vi "Launch Main.vi"(8 "error in":errorcluster, 9 "Name":string, 10 "Path":path=path "C:/Users/Public/Documents/Development/AppDemo", 11 "notifier in":refnum<notifier>) -> (0 "error out":errorcluster, 2 "Main Enqueuer":refnum<class "Message Enqueuer.lvclass">, 3 "notifier out":refnum<notifier>)   [LabVIEW 2023, in "Main.lvlib"]
uses:
  Library/Main.lvlib
  Library/Main.lvclass
  builds/Framework/Panel Manager.lvlibp/Panel/Window Position/Reference Position/Alignment.ctl
  builds/Framework/Panel Manager.lvlibp/Panel/Window Position/Reference Position/Horizontal Alignment.ctl
  builds/Framework/Panel Manager.lvlibp/Panel/Window Position/Reference Position/Vertical Alignment.ctl
  builds/Framework/Panel Manager.lvlibp/Panel/Window Position/Reference Position/Ref Display/Ref Display.lvclass
  builds/Framework/Engine.lvlibp/Engine/Accessors/Write IsRoot.vi
  builds/Framework/Engine.lvlibp/Engine/Accessors/Write Application Path.vi
  builds/Framework/Panel Manager.lvlibp/Panel Actor/Panel Actor/Launch Root Panel Window.vi
  builds/Framework/Panel Manager.lvlibp/Panel/Window Position/Reference Position/Ref Display/Ref Display.vi
  builds/Framework/Panel Manager.lvlibp/Library/Panel Actor.lvclass
  builds/Framework/Panel Manager.lvlibp/Panel/Panel.lvlib
  builds/Framework/Panel Manager.lvlibp/Panel/Window Position/Reference Position/Reference Position.lvclass
  builds/Framework/Actor Framework.lvlibp/1abvi3w/vi.lib/ActorFramework/Message Enqueuer/Message Enqueuer.lvclass
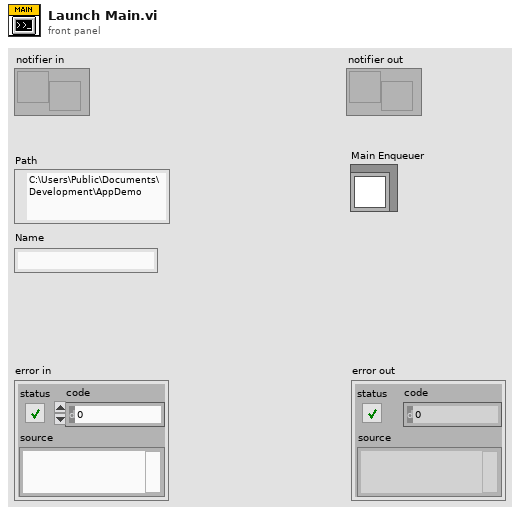
[diagram p1: front panel]
types:
  T1 = typedef "Panel Manager.lvlibp/Panel.lvlib/Reference Position.lvclass/Alignment.ctl" = cluster{"Horizontal":T2, "Vertical":T3}
  T2 = typedef "Panel Manager.lvlibp/Panel.lvlib/Reference Position.lvclass/Horizontal Alignment.ctl" = enum16{"Left", "Center", "Right"}
  T3 = typedef "Panel Manager.lvlibp/Panel.lvlib/Reference Position.lvclass/Vertical Alignment.ctl" = enum16{"Top", "Center", "Bottom"}
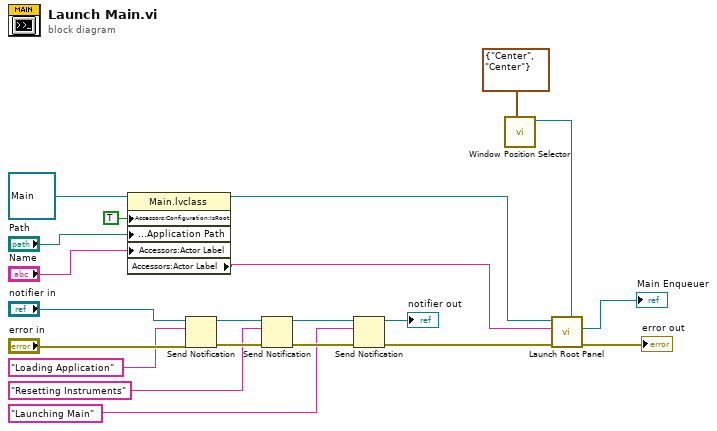
[diagram p0: block diagram]
diagram:
  n1 = property class="Main.lvclass"(reference=refnum<class "Main.lvclass"> refnum ("Main.lvlib:Main.lvclass"), "Accessors:Configuration:IsRoot"=TRUE ("Engine:Configuration:IsRoot"), "Accessors:Configuration:Application Path"="Path", "Accessors:Actor Label"="Name") -> (reference out=w20:refnum<class "Main.lvclass">, "Accessors:Actor Label"=w1:string)  [unwired: 1 in, 1 out]
  n2 = Send Notification(notification="Loading Application", notifier="notifier in", error in (no error)="error in") -> (notifier out=w10:refnum<notifier>, error out=w11:errorcluster)
  n3 = Send Notification(notification="Resetting Instruments", notifier=w10, error in (no error)=w11) -> (notifier out=w7:refnum<notifier>, error out=w8:errorcluster)
  n4 = Send Notification(notification="Launching Main", notifier=w7, error in (no error)=w8) -> (notifier out=→"notifier out":refnum<notifier>, error out=w4:errorcluster)
  n5 = call-poly "Window Position Selector.vi"("Alignment"=T1 {"Horizontal"=enum."Center", "Vertical"=enum."Center"}) -> ("Ref Display out"=w18:refnum<class "Ref Display.lvclass">)  [unwired: 9 in, 1 out]
  n6 = call-poly "Launch Root Panel.vi"("Window Position (Maximize First Call)"=w18, "Error In"=w4, "Title"=w1, "Panel Actor in"=w20) -> ("Error Out"=→"error out":errorcluster, "Actor's Enqueuer"=→"Main Enqueuer":refnum<class "Message Enqueuer.lvclass">)  [unwired: 6 in]
